vi "GetEdge DetectionResultNames.vi"(7 "ProjectName":string="Prj", 10 "Analysis_Edge Detection_Parameter":T3={"Edge Options"={"Edge Polarity"=0, "Kernel Size"=3, "Width"=5, "Minimum Edge Strength"=10.0, "Interpolation Type"=1, "Data Processing Method"=0}, "Process"=2, "Number of Matches Requested"=1, "ROI Descriptor"={"Global Rectangle"=[], "Contours"=[]}} {"Process" items=["Get First Edge", "Get First + Last Edge", "Get All Edges", "Get Best Edge"]; "Edge Options"."Data Processing Method" items=["Average", "Median"]; "Edge Options"."Interpolation Type" items=["Zero Order"=0, "Bilinear"=1, "Bilinear Fixed"=4]; "Edge Options"."Minimum Edge Strength" min=0.0 max=255.0 format="%.2g"; "Edge Options"."Width" min=1 step=2; "Edge Options"."Kernel Size" min=3 step=2; "Edge Options"."Edge Polarity" items=["All Edges", "Rising Edges", "Falling Edges"]}, 11 "ROI_Name":string="ROI1") -> (3 "ResultNames":string[](array[string]))   [LabVIEW 2019]
uses:
  Controls/Edge Detection/Analysis_Edge Detection_Parameter.ctl
  Controls/Edge Detection/Analysis_Edge Detection_Result.ctl
  <vilib>/vision/Measure.llb/Edge New.ctl
panel:
  in  "Analysis_Edge Detection_Result":T1 {"Edge Information"."Distance (Real-World)" format="%.2f"; "Edge Information"."Location (Real-World)"."Y" format="%.2g"; "Edge Information"."Location (Real-World)"."X" format="%.2f"; "Edge Information"."Noise" format="%.2f"; "Edge Information"."Location (Pixel)"."Y" format="%.2g"; "Edge Information"."Location (Pixel)"."X" format="%.2f"; "Edge Information"."Strength" format="%.2f"; "Edge Information"."Distance (Pixel)" format="%.2f"}
  out "error out":errorcluster
  in  "error in (no error)":errorcluster
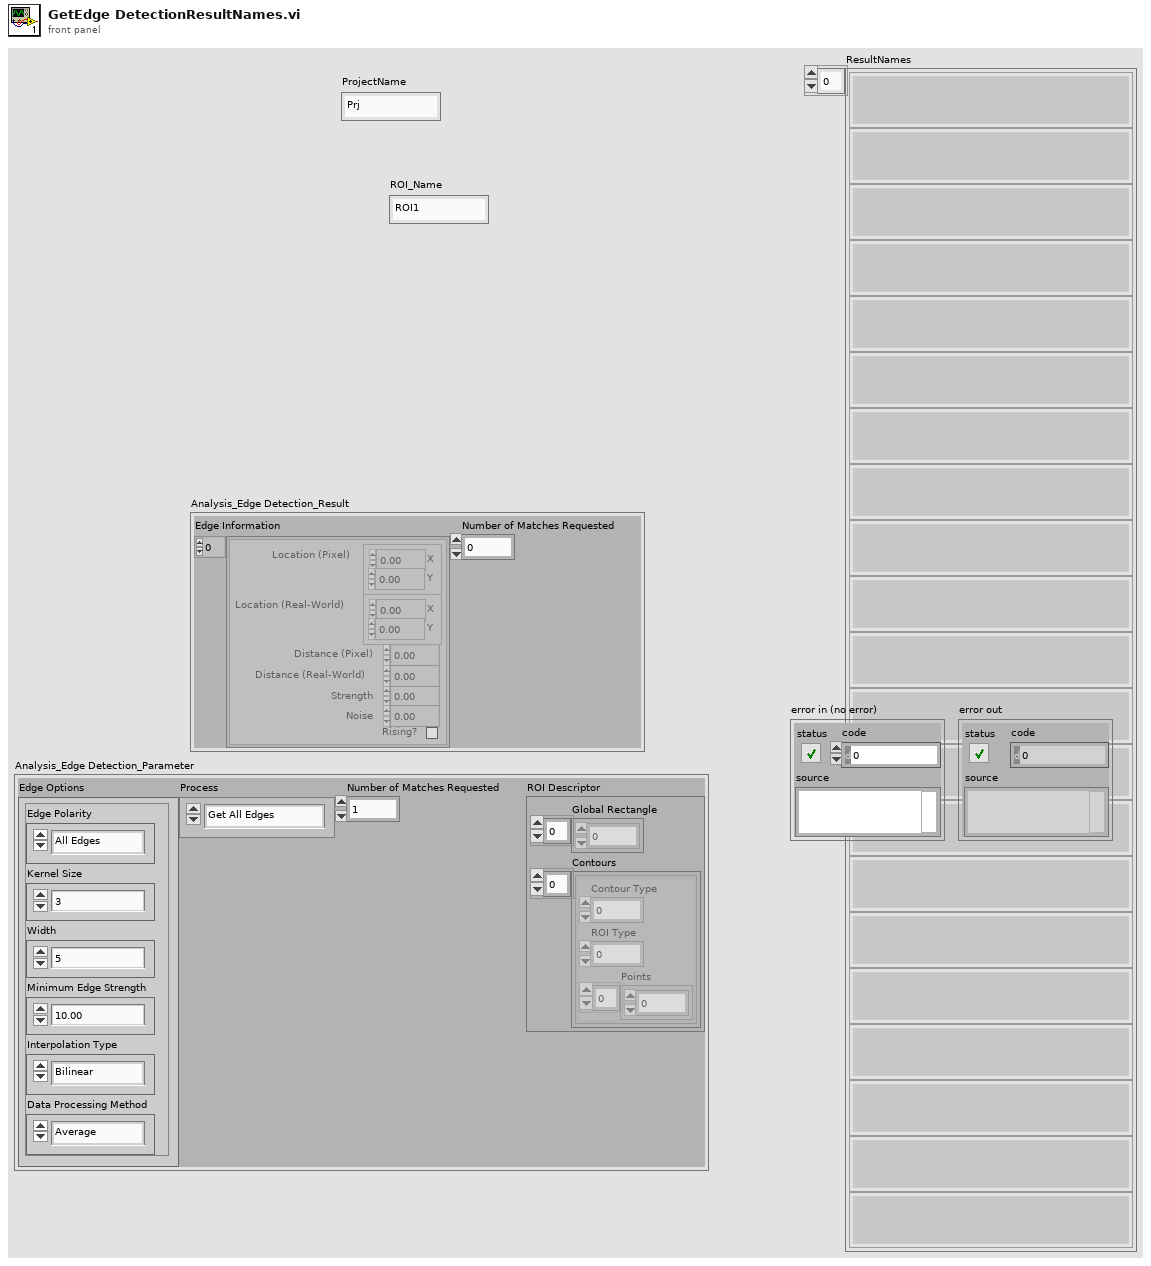
[diagram p1: front panel]
types:
  T1 = typedef "Analysis_Edge Detection_Result.ctl" = cluster{"Edge Information":T2[], "Number of Matches Requested":i32}
  T2 = typedef "Edge New.ctl" = cluster{"Location (Pixel)":cluster{"X":sgl, "Y":sgl}, "Location (Real-World)":cluster{"X":sgl, "Y":sgl}, "Distance (Pixel)":dbl, "Distance (Real-World)":dbl, "Strength":dbl, "Noise":dbl, "Rising?":bool}
  T3 = typedef "Analysis_Edge Detection_Parameter.ctl" = cluster{"Edge Options":cluster{"Edge Polarity":u16, "Kernel Size":u32, "Width":u32, "Minimum Edge Strength":dbl, "Interpolation Type":u16, "Data Processing Method":u16}, "Process":u16, "Number of Matches Requested":i32, "ROI Descriptor":cluster{"Global Rectangle":i32[], "Contours":cluster{"Contour Type":u32, "ROI Type":u32, "Points":i32[]}[]}}
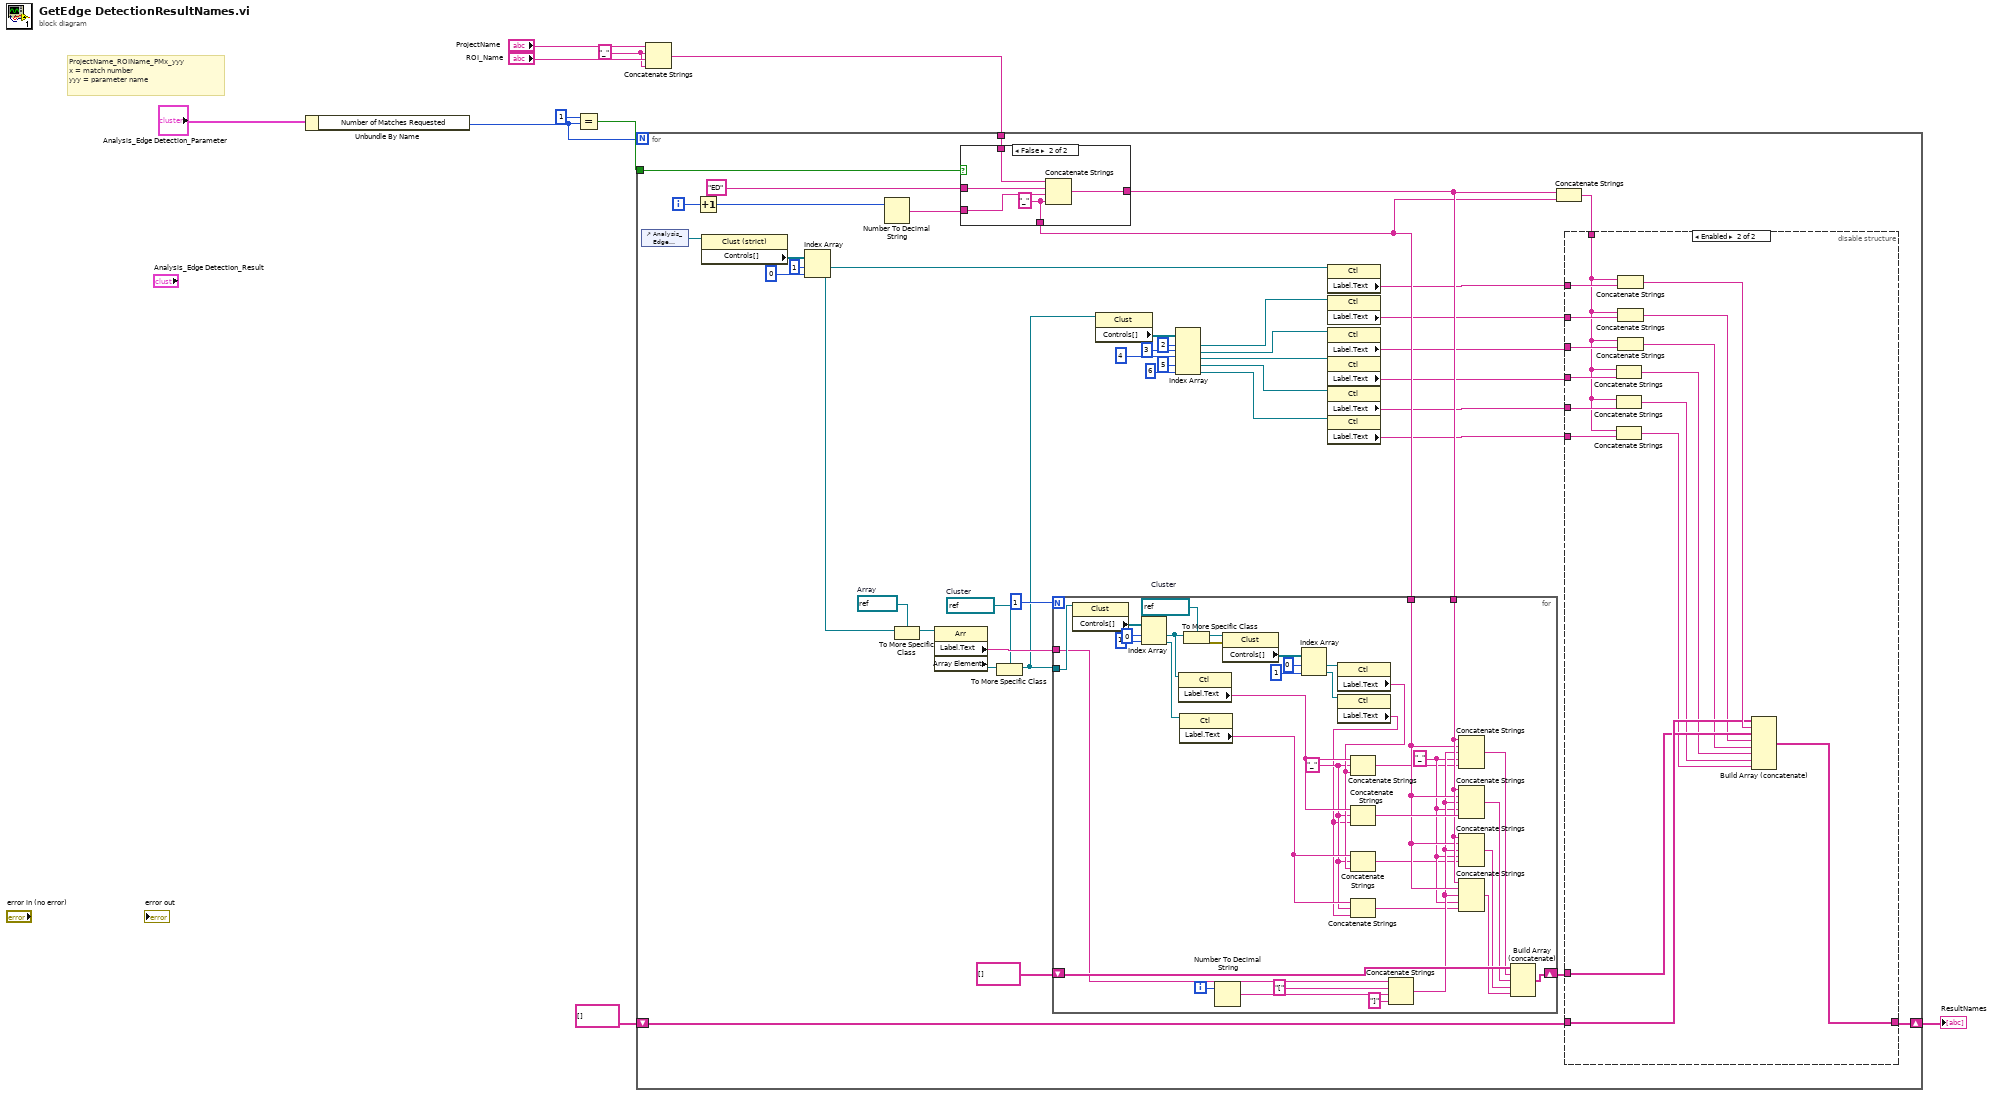
[diagram p0: block diagram]
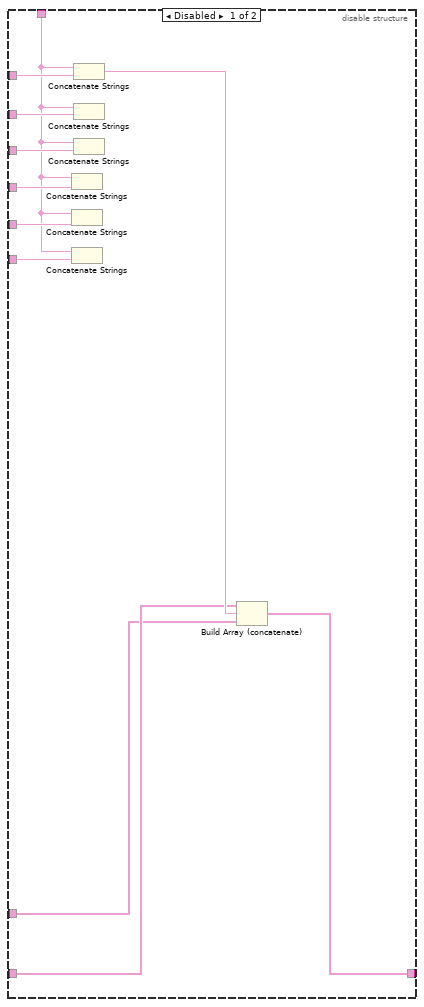
[diagram p2: hidden frame]
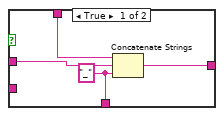
[diagram p3: hidden frame]
diagram:
  w7 = "_" ("string")
  # "ProjectName_ROIName_PMx_yyy\nx = match number\nyyy = parameter name"
  n1 = Unbundle By Name("Analysis_Edge Detection_Parameter") -> ("Number of Matches Requested"=w2:i32)
  n2 = Equal?(x=1, y=w2) -> (x = y?=w3:bool)
  n3 = Concatenate Strings("ProjectName", w7, "ROI_Name", w7) -> (w6:string)
  n4 = for {
    N: w2 -> [_]
    tunnel: w6 -> [w51]
    shift-right: [w38] -> w4
    shift-left: string[] [] -> [w47]
    tunnel: w3 -> [w52]
    i -> [w48]
    w33 = refnum<vi> refnum  # Cluster
    w35 = refnum<vi> refnum  # Array
    n5 = control-ref of="Analysis_Edge Detection_Result"() -> (w11:refnum<vi>)
    n6 = Increment(x=w48) -> (x+1=w53:i32)
    n7 = property class="Clust (strict)"(reference=w11) -> ("Controls[]"=w37:refnum<vi>[])  [unwired: 1 in, 2 out]
    n8 = Index Array(array=w37, index #1=1 ("index"), index #2=0 ("index")) -> (element #1=w31:refnum<vi>, element #2=w29:refnum<vi>)
    n9 = Number To Decimal String(number=w53) -> (decimal integer string=w50:string)  [unwired: 1 in]
    n10 = To More Specific Class(target class=w35, reference=w29) -> (specific class reference=w34:refnum<vi>)  [unwired: 1 in, 1 out]
    n11 = property class="Arr"(reference=w34) -> ("Label.Text"=w46:string, "Array Element"=w32:refnum<vi>)  [unwired: 1 in, 2 out]
    n12 = case shown="False" w52 {
      tunnel: w51 -> [w122 w127]
      tunnel: w50 -> [_ w125]
      tunnel: [w121 w126] -> w42
      tunnel: "ED" ("string") -> [w120 w124]
      tunnel: [w119 w123] -> w41
      frame True {
        w119 = "_" ("string")
        n13 = Concatenate Strings(w122, w120, w119) -> (w121:string)
      }
      frame False {
        w123 = "_" ("string")
        n14 = Concatenate Strings(w127, w124, w125, w123) -> (w126:string)
      }
    }
    n15 = To More Specific Class(target class=w33, reference=w32) -> (specific class reference=w28:refnum<vi>)  [unwired: 1 in, 1 out]
    n16 = for {
      N: 1 -> [_]
      tunnel: w46 -> [w112]
      tunnel: w28 -> [w118]
      tunnel: w42 -> [w91]
      tunnel: w41 -> [w90]
      shift-right: [w114] -> w43
      shift-left: string[] [] -> [w117]
      i -> [w113]
      w84 = "_" ("string")
      w105 = refnum<vi> refnum  # Cluster
      w88 = "_" ("string")
      n17 = property class="Clust"(reference=w118) -> ("Controls[]"=w108:refnum<vi>[])  [unwired: 1 in, 2 out]
      n18 = Index Array(array=w108, index #1=0 ("index"), index #2=1 ("index")) -> (element #1=w97:refnum<vi>, element #2=w96:refnum<vi>)
      n19 = property class="Ctl"(reference=w97) -> ("Label.Text"=w95:string)  [unwired: 1 in, 2 out]
      n20 = property class="Ctl"(reference=w96) -> ("Label.Text"=w86:string)  [unwired: 1 in, 2 out]
      n21 = To More Specific Class(target class=w105, reference=w97) -> (specific class reference=w104:refnum<vi>, error out=w103:errorcluster)  [unwired: 1 in]
      n22 = Number To Decimal String(number=w113) -> (decimal integer string=w110:string)  [unwired: 1 in]
      n23 = property class="Clust"(reference=w104, error in=w103) -> ("Controls[]"=w102:refnum<vi>[])  [unwired: 2 out]
      n24 = Index Array(array=w102, index #1=0 ("index"), index #2=1 ("index")) -> (element #1=w99:refnum<vi>, element #2=w98:refnum<vi>)
      n25 = property class="Ctl"(reference=w99) -> ("Label.Text"=w85:string)  [unwired: 1 in, 2 out]
      n26 = property class="Ctl"(reference=w98) -> ("Label.Text"=w83:string)  [unwired: 1 in, 2 out]
      n27 = Concatenate Strings(w95, w84, w85) -> (w87:string)
      n28 = Concatenate Strings(w95, w84, w83) -> (w94:string)
      n29 = Concatenate Strings(w86, w84, w85) -> (w82:string)
      n30 = Concatenate Strings(w86, w84, w83) -> (w81:string)
      n31 = Concatenate Strings(w112, "[" ("string"), w110, "]" ("string")) -> (w89:string)
      n32 = Concatenate Strings(w91, w90, w89, w88, w87) -> (w116:string)
      n33 = Concatenate Strings(w91, w90, w89, w88, w94) -> (w115:string)
      n34 = Concatenate Strings(w91, w90, w89, w88, w82) -> (w93:string)
      n35 = Concatenate Strings(w91, w90, w89, w88, w81) -> (w92:string)
      n36 = Build Array (concatenate)(w117, w116, w115, w93, w92) -> (w114:string[])
    }
    n37 = property class="Clust"(reference=w28) -> ("Controls[]"=w27:refnum<vi>[])  [unwired: 1 in, 2 out]
    n38 = Index Array(array=w27, index #1=2 ("index"), index #2=3 ("index"), index #3=4 ("index"), index #4=5 ("index"), index #5=6 ("index")) -> (element #1=w21:refnum<vi>, element #2=w19:refnum<vi>, element #3=w18:refnum<vi>, element #4=w15:refnum<vi>, element #5=w14:refnum<vi>)
    n39 = property class="Ctl"(reference=w31) -> ("Label.Text"=w40:string)  [unwired: 1 in, 2 out]
    n40 = property class="Ctl"(reference=w21) -> ("Label.Text"=w20:string)  [unwired: 1 in, 2 out]
    n41 = property class="Ctl"(reference=w19) -> ("Label.Text"=w17:string)  [unwired: 1 in, 2 out]
    n42 = property class="Ctl"(reference=w18) -> ("Label.Text"=w16:string)  [unwired: 1 in, 2 out]
    n43 = property class="Ctl"(reference=w15) -> ("Label.Text"=w13:string)  [unwired: 1 in, 2 out]
    n44 = property class="Ctl"(reference=w14) -> ("Label.Text"=w12:string)  [unwired: 1 in, 2 out]
    n45 = Concatenate Strings(w42, w41) -> (w39:string)
    n46 = disable-structure shown="Enabled" {
      disable-tunnel: w47 -> [w55 w71]
      disable-tunnel: w43 -> [w54 w70]
      disable-tunnel: w40 -> [w63 w79]
      disable-tunnel: w20 -> [w61 w77]
      disable-tunnel: w16 -> [w59 w75]
      disable-tunnel: w13 -> [w58 w74]
      disable-tunnel: w39 -> [w56 w72]
      disable-tunnel: [w64 w80] -> w38
      disable-tunnel: w12 -> [w57 w73]
      disable-tunnel: w17 -> [w60 w76]
      frame Disabled {
        n47 = Concatenate Strings(w56, w59) -> ()  [unwired: 1 out]
        n48 = Concatenate Strings(w56, w58) -> ()  [unwired: 1 out]
        n49 = Concatenate Strings(w56, w57) -> ()  [unwired: 1 out]
        n50 = Concatenate Strings(w56, w63) -> (w62:string)
        n51 = Concatenate Strings(w56, w61) -> ()  [unwired: 1 out]
        n52 = Concatenate Strings(w56, w60) -> ()  [unwired: 1 out]
        n53 = Build Array (concatenate)(w55, w62, w54) -> (w64:string[])
      }
      frame Enabled {
        n54 = Concatenate Strings(w72, w75) -> (w67:string)
        n55 = Concatenate Strings(w72, w74) -> (w66:string)
        n56 = Concatenate Strings(w72, w73) -> (w65:string)
        n57 = Concatenate Strings(w72, w79) -> (w78:string)
        n58 = Concatenate Strings(w72, w77) -> (w69:string)
        n59 = Concatenate Strings(w72, w76) -> (w68:string)
        n60 = Build Array (concatenate)(w71, w78, w70, w69, w68, w67, w66, w65) -> (w80:string[])
      }
    }
  }
  "ResultNames" <- w4
